vi "Arduino_Opta.vi"(8 "error in":errorcluster, 10 "On/Off":T1=enum."On", 11 "Parameters":T2) -> (0 "error out":errorcluster, 2 "Standard Output":string, 3 "Output":bool)   [LabVIEW 2025]
uses:
  Control/Parameters.ctl
  Control/Trigger.ctl
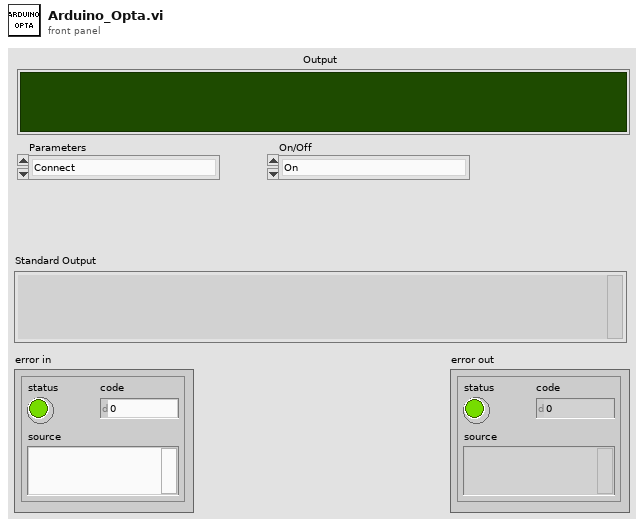
[diagram p1: front panel]
types:
  T1 = typedef "Trigger.ctl" = enum16{"", "On", "Off"}
  T2 = typedef "Parameters.ctl" = enum16{"Connect", "Disconnect", "Main_Valve_EN", "Valve1_EN", "Valve2_EN", "Valve3_EN", "Valve4_EN", "Valve5_EN", "Fix_Power_EN", "Spare1", "Spare2", "Spare3", "Spare4", "Spare5"}
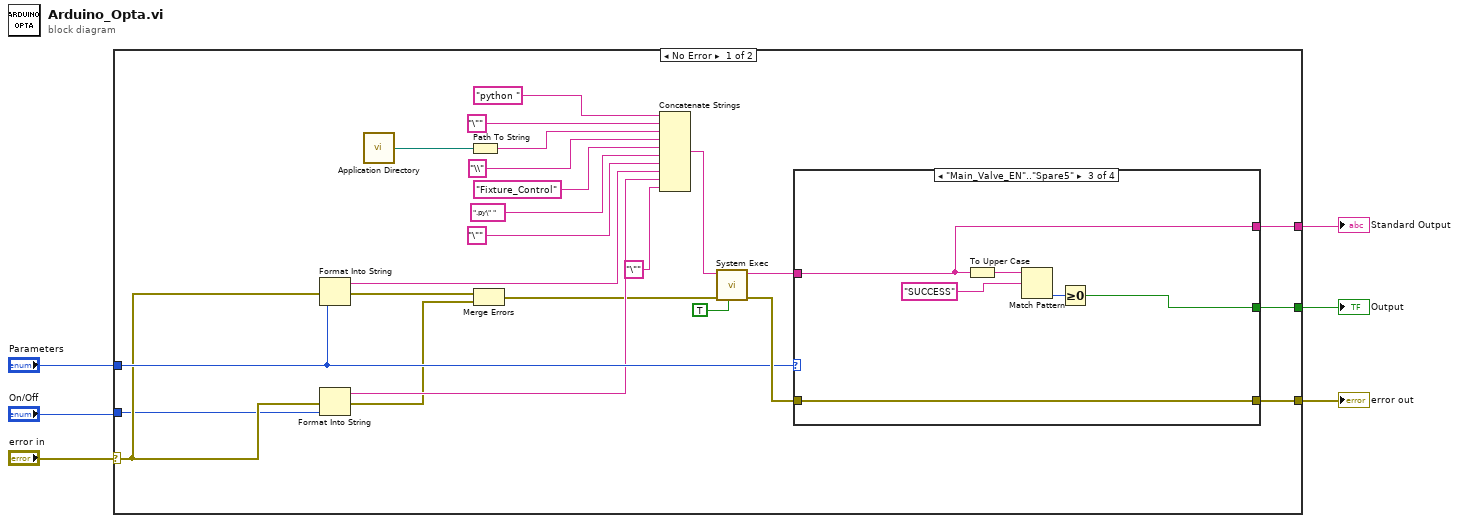
[diagram p0: block diagram]
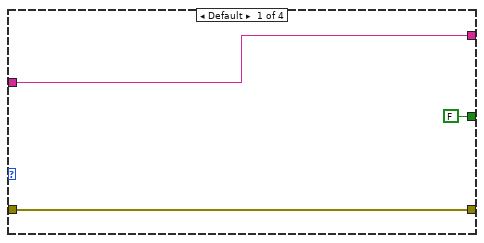
[diagram p2: hidden frame]
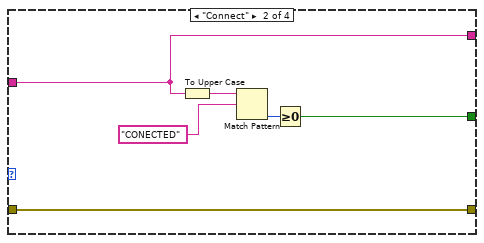
[diagram p3: hidden frame]
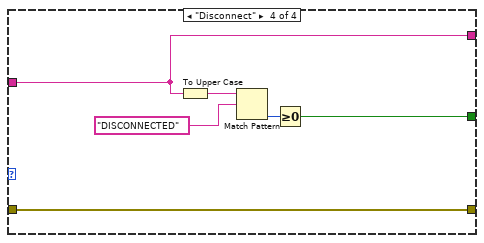
[diagram p4: hidden frame]
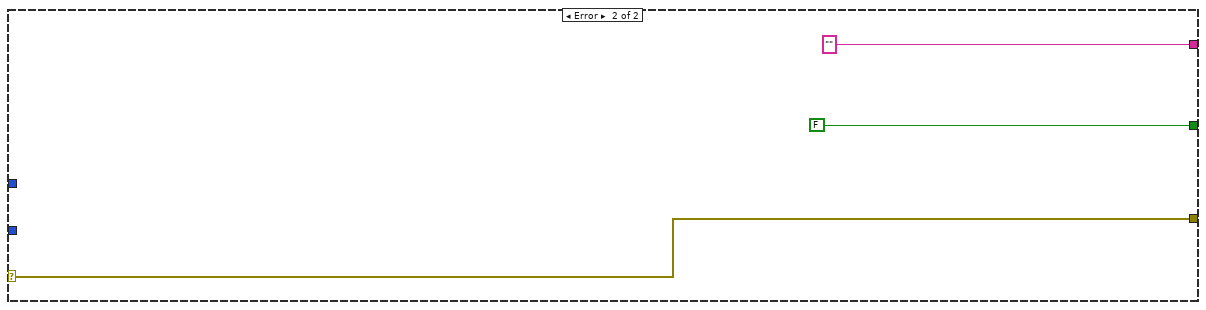
[diagram p5: hidden frame]
diagram:
  n1 = case shown="No Error" "error in" {
    selector: "error in" -> [w15 w54]
    tunnel: [w26 w54] -> w5
    tunnel: "Parameters" -> [w25 _]
    tunnel: [w23 "" ("standard output")] -> w4
    tunnel: [w24 FALSE] -> w3
    tunnel: "On/Off" -> [w14 _]
    frame No Error {
      n2 = Format Into String(error in=w15, w25) -> (resulting string=w13:string, error out=w9:errorcluster)  [unwired: 2 in]
      n3 = Format Into String(error in=w15, w14) -> (resulting string=w12:string, error out=w8:errorcluster)  [unwired: 2 in]
      n4 = call <vilib>:"Application Directory.vi"() -> ("Application Directory"=w30:path)
      n5 = Path To String(path=w30) -> (string=w29:string)
      n6 = Merge Errors(w9, w8) -> (w7:errorcluster)
      n7 = Concatenate Strings("python " ("string"), "\"" ("string"), w29, "\\" ("string"), "Fixture_Control" ("string"), ".py\" " ("string"), "\"" ("string"), w13, w12, "\"" ("string")) -> (w17:string)
      n8 = call <vilib>:"System Exec.vi"("run minimized? (F)"=TRUE, "error in (no error)"=w7, "command line"=w17) -> ("error out"=w27:errorcluster, "standard output"=w22:string)  [unwired: 5 in, 2 out]
      n9 = case shown="\"Main_Valve_EN\"..\"Spare5\"" w25 {
        tunnel: [FALSE w36 w42 w48] -> w24
        tunnel: w27 -> [w33 w37 w43 w49]
        tunnel: [w33 w37 w43 w49] -> w26
        tunnel: [w32 w35 w41 w47] -> w23
        tunnel: w22 -> [w32 w35 w41 w47]
        frame Default {
        }
        frame "Connect" {
          n10 = To Upper Case(1:w35) -> (0:w34:string)
          n11 = Match Pattern(string=w34, regular expression="CONECTED") -> (offset past match=w38:i32)  [unwired: 1 in, 3 out]
          n12 = Greater Or Equal To 0?(x=w38) -> (x >= 0?=w36:bool)
        }
        frame "Main_Valve_EN".."Spare5" {
          n13 = To Upper Case(1:w41) -> (0:w40:string)
          n14 = Match Pattern(string=w40, regular expression="SUCCESS") -> (offset past match=w44:i32)  [unwired: 1 in, 3 out]
          n15 = Greater Or Equal To 0?(x=w44) -> (x >= 0?=w42:bool)
        }
        frame "Disconnect" {
          n16 = To Upper Case(1:w47) -> (0:w46:string)
          n17 = Match Pattern(string=w46, regular expression="DISCONNECTED") -> (offset past match=w50:i32)  [unwired: 1 in, 3 out]
          n18 = Greater Or Equal To 0?(x=w50) -> (x >= 0?=w48:bool)
        }
      }
    }
    frame Error {
    }
  }
  "error out" <- w5
  "Standard Output" <- w4
  "Output" <- w3
